vi "lfield_stream_frames.vi"(8 "error in (no error)":errorcluster, 9 "stop_image_stream":refnum<queue>, 10 "stop_stream_queue":refnum<queue>, 11 "lightfield_class in":refnum<class "lightfield_class.lvclass">) -> (0 "error out":errorcluster, 3 "lightfield_class out":refnum<class "lightfield_class.lvclass">)   [LabVIEW 2015, in "lightfield_class.lvclass"]
uses:
  lightfield_class.lvclass
  lightfield_class.lvclass/lightfield_class.ctl
  lightfield-automation-labview/LightField Automation.lvclass
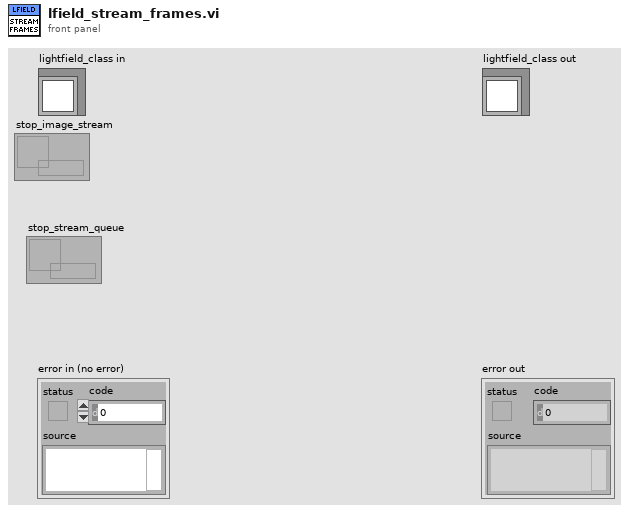
[diagram p1: front panel]
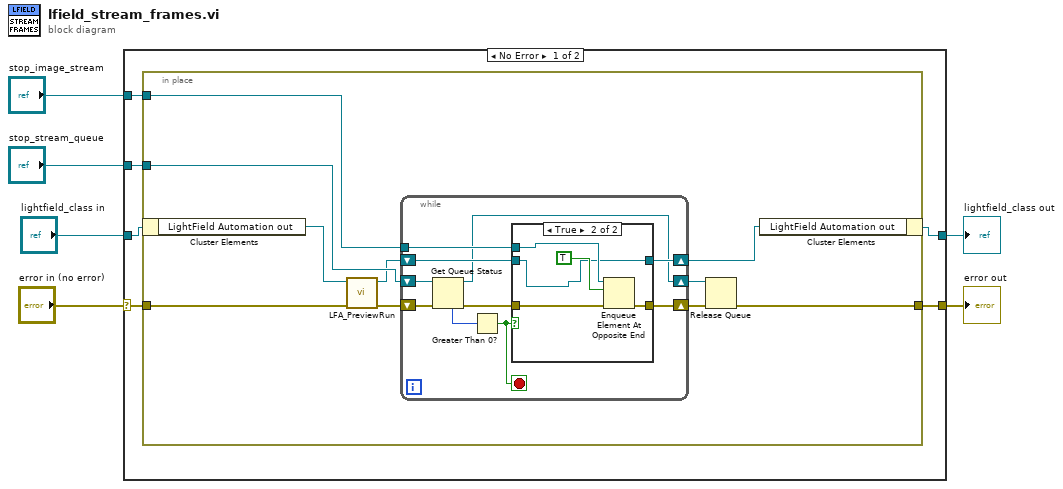
[diagram p0: block diagram]
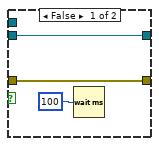
[diagram p2: hidden frame]
diagram:
  n1 = case shown="No Error" "error in (no error)" {
    selector: "error in (no error)" -> [w11 w42]
    tunnel: [w8 w42] -> w5
    tunnel: [w10 w41] -> w3
    tunnel: "lightfield_class in" -> [w12 w41]
    tunnel: "stop_stream_queue" -> [w9 _]
    tunnel: "stop_image_stream" -> [w7 _]
    frame No Error {
      n2 = in-place {
        in-place-border: w11 -> [w18]
        in-place-border: w9 -> [w22]
        in-place-border: [w15] -> w8
        in-place-border: w7 -> [w17]
        n3 = in-place-cluster #1(w12) -> ("LightField Automation out"=w21:refnum<class "LightField Automation.lvclass">)
        n4 = call "LFA_PreviewRun.vi"("error in (no error)"=w18, "LightField Automation in"=w21) -> ("error out"=w19:errorcluster, "LightField Automation out"=w20:refnum<class "LightField Automation.lvclass">)  [unwired: 8 in]
        n5 = while {
          shift-right: [w30] -> w16
          shift-left: w20 -> [w31]
          shift-right: [w29] -> w13
          shift-left: w19 -> [w27]
          tunnel: w17 -> [w28]
          shift-right: [w24] -> w14
          shift-left: w22 -> [w25]
          stop <- w32 stop-if-true
          n6 = Get Queue Status(queue=w25, error in (no error)=w27) -> (queue out=w24:refnum<queue>, error out=w26:errorcluster, # elements in queue=w23:i32)  [unwired: 1 in, 5 out]
          n7 = Greater Than 0?(x=w23) -> (x > 0?=w32:bool)
          n8 = case shown="True" w32 {
            tunnel: w31 -> [w35 w36]
            tunnel: [w35 w36] -> w30
            tunnel: w26 -> [w34 w37]
            tunnel: [w34 w40] -> w29
            tunnel: w28 -> [_ w39]
            frame False {
              n9 = Wait (ms)(milliseconds to wait=u32 100) -> ()  [unwired: 1 out]
            }
            frame True {
              n10 = Enqueue Element At Opposite End(queue=w39, element=TRUE ("notification"), error in (no error)=w37) -> (error out=w40:errorcluster)  [unwired: 1 in, 2 out]
            }
          }
        }
        n11 = Release Queue(queue=w14, error in (no error)=w13) -> (error out=w15:errorcluster)  [unwired: 1 in, 2 out]
        n12 = in-place-cluster #1("LightField Automation out"=w16) -> (w10:refnum<class "lightfield_class.lvclass">)
      }
    }
    frame Error {
    }
  }
  "error out" <- w5
  "lightfield_class out" <- w3
